vi "Write String Array Units.vi"(8 "Error In":errorcluster, 9 "Heating Value (BTU/ft³)":dbl=1000.0 min=900.0 max=2600.0 step=1.0, 10 "Header Array":string[](array[string]), 11 "Data Cluster":T1) -> (0 "Error Out":errorcluster, 3 "String Data":string[][](array[string]))   [LabVIEW 2019]
uses:
  Data Cluster.ctl
  Trunk/Utility/Type Definitions/UTILITY Notifier.ctl
panel:
  in  "Header Array Debug":string[](array[string])=["Time Stamp", "Absolute Pressure", "Gauge/Diff. Pressure", "BarometricPressure", "Temperature", "Uncorrected", "Corrected", "Totalizer", "Tot. Timer", "Tot. Avg. Flow", "Tot. Peak Flow", "Gas Selected"]
  # "Totalizer Timer"
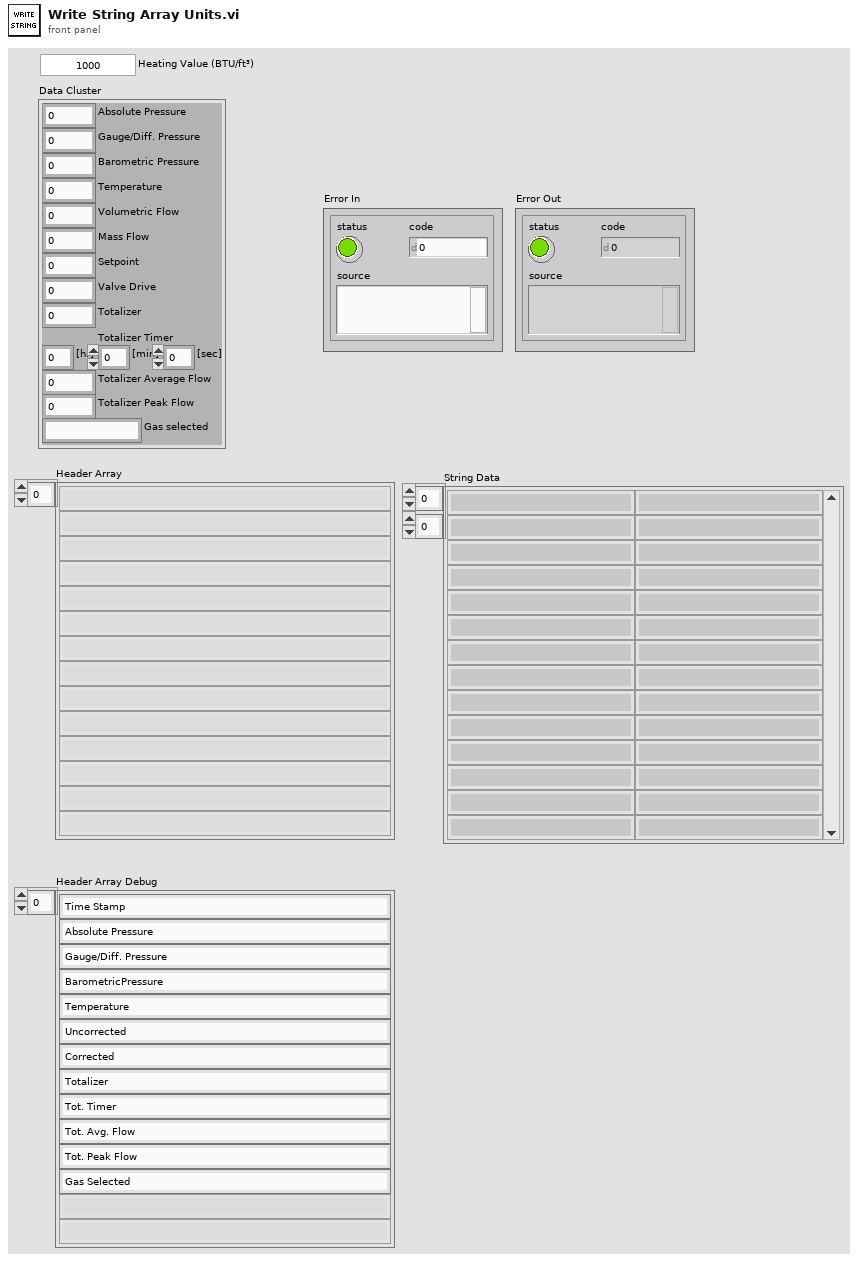
[diagram p1: front panel]
types:
  T1 = typedef "Data Cluster.ctl" = cluster{"Absolute Pressure":dbl, "Gauge/Diff. Pressure":dbl, "Barometric Pressure":dbl, "Temperature":dbl, "Volumetric Flow":dbl, "Mass Flow":dbl, "Setpoint":dbl, "Valve Drive":dbl, "Totalizer":dbl, "[hr]":dbl, "[min]":dbl, "[sec]":dbl, "Totalizer Average Flow":dbl, "Totalizer Peak Flow":dbl, "Gas selected":string}
  T2 = typedef "UTILITY Notifier.ctl" = enum16{"Set", "Read", "Release Ref"}
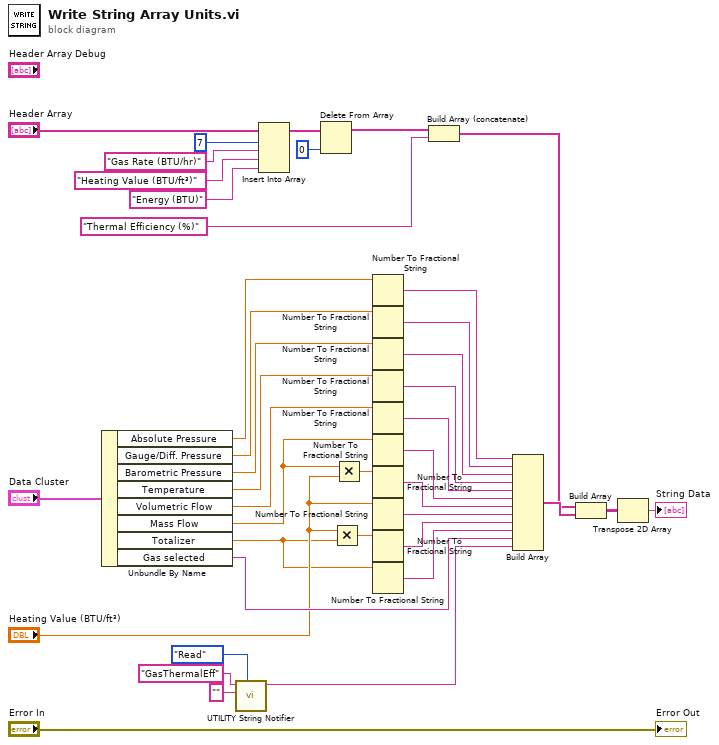
[diagram p0: block diagram]
diagram:
  n1 = Unbundle By Name("Data Cluster") -> ("Absolute Pressure"=w34:dbl, "Gauge/Diff. Pressure"=w35:dbl, "Barometric Pressure"=w36:dbl, "Temperature"=w37:dbl, "Volumetric Flow"=w38:dbl, "Mass Flow"=w22:dbl, "Totalizer"=w9:dbl, "Gas selected"=w26:string)
  n2 = call "UTILITY String Notifier.vi"("Status"=UTILITY_Notifier."Read", "Set Status"="", "name (unnamed)"="GasThermalEff") -> ("latest notification"=w5:string)  [unwired: 7 in, 1 out]
  n3 = Insert Into Array(array="Header Array", index=7, new element #1="Gas Rate (BTU/hr)" ("new element/subarray"), new element #2="Heating Value (BTU/ft³)" ("new element/subarray"), new element #3="Energy (BTU)" ("new element/subarray")) -> (w17:string[])
  n4 = Delete From Array(array=w17, index=0) -> (array with subset deleted=w4:string[])  [unwired: 1 in, 1 out]
  n5 = Multiply(x="Heating Value (BTU/ft³)", y=w9) -> (x*y=w15:dbl)
  n6 = Multiply(x=w22, y="Heating Value (BTU/ft³)") -> (x*y=w21:dbl)
  n7 = Number To Fractional String(number=w34) -> (F-format string=w32:string)  [unwired: 3 in]
  n8 = Number To Fractional String(number=w35) -> (F-format string=w31:string)  [unwired: 3 in]
  n9 = Number To Fractional String(number=w36) -> (F-format string=w30:string)  [unwired: 3 in]
  n10 = Number To Fractional String(number=w37) -> (F-format string=w29:string)  [unwired: 3 in]
  n11 = Number To Fractional String(number=w38) -> (F-format string=w28:string)  [unwired: 3 in]
  n12 = Number To Fractional String(number=w22) -> (F-format string=w27:string)  [unwired: 3 in]
  n13 = Number To Fractional String(number=w21) -> (F-format string=w20:string)  [unwired: 3 in]
  n14 = Number To Fractional String(number="Heating Value (BTU/ft³)") -> (F-format string=w16:string)  [unwired: 3 in]
  n15 = Number To Fractional String(number=w15) -> (F-format string=w12:string)  [unwired: 3 in]
  n16 = Number To Fractional String(number=w9) -> (F-format string=w11:string)  [unwired: 3 in]
  n17 = Build Array (concatenate)(w4, "Thermal Efficiency (%)" ("new element/subarray")) -> (w3:string[])
  n18 = Build Array(w32, w31, w30, w29, w28, w27, w20, w16, w12, w11, w26, w5) -> (w25:string[])
  n19 = Build Array(w3, w25) -> (w39:string[][])
  n20 = Transpose 2D Array(2D array=w39) -> (transposed array=→"String Data":string[][])
  "Error Out" <- "Error In"
